vi "Update State.vi"(8 "error in (no error)":errorcluster, 11 "BiStableShutter in":refnum<class "BiStableShutter.lvclass">) -> (0 "error out":errorcluster, 3 "BiStableShutter out":refnum<class "BiStableShutter.lvclass">)   [LabVIEW 2016, in "BiStableShutter.lvclass"]
uses:
  BiStableShutter.lvclass
  Controls/Shutter States.ctl
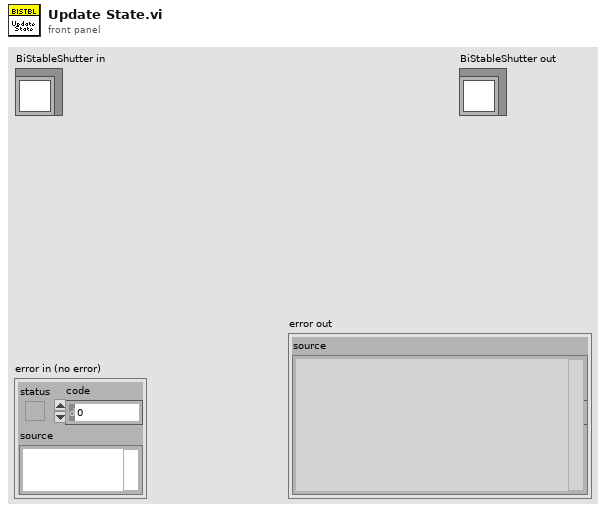
[diagram p1: front panel]
types:
  T1 = typedef "Shutter States.ctl" = enum16{"Open", "Close", "Wait", "Off", "Arm", "Idle"}
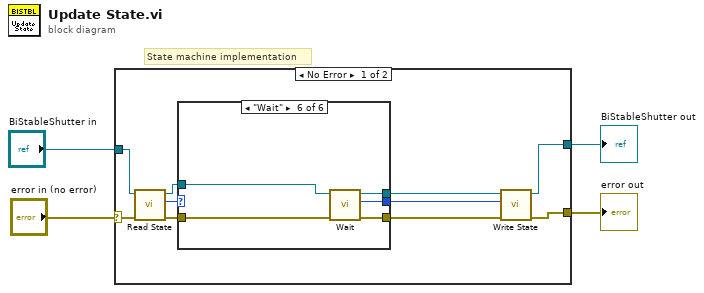
[diagram p0: block diagram]
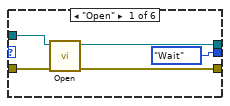
[diagram p2: hidden frame]
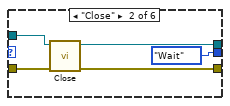
[diagram p3: hidden frame]
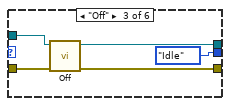
[diagram p4: hidden frame]
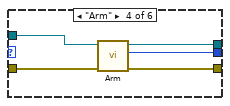
[diagram p5: hidden frame]
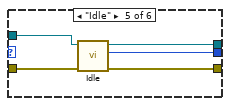
[diagram p6: hidden frame]
diagram:
  # "State machine implementation"
  n1 = case shown="No Error" "error in (no error)" {
    selector: "error in (no error)" -> [w5 w46]
    tunnel: [w14 w45] -> w4
    tunnel: [w12 w46] -> w3
    tunnel: "BiStableShutter in" -> [w9 w45]
    frame No Error {
      n2 = call-dynamic "Read State.vi"("error in (no error)"=w5, "Shutter in"=w9) -> ("error out"=w7:errorcluster, "State"=w6:T1, "Shutter out"=w8:refnum<class "BiStableShutter.lvclass">)  [unwired: 7 in]
      n3 = case shown="\"Wait\"" w6 {
        tunnel: w8 -> [w18 w24 w27 w34 w39 w44]
        tunnel: w7 -> [w19 w23 w29 w30 w38 w43]
        tunnel: [w16 w21 w28 w31 w35 w40] -> w13
        tunnel: [w15 w22 w26 w33 w36 w42] -> w10
        tunnel: [Shutter_States."Wait" ("State") Shutter_States."Wait" ("f") Shutter_States."Idle" ("State") w32 w37 w41] -> w11
        frame "Open" {
          n4 = call-dynamic "Open.vi"("error in (no error)"=w19, "BiStableShutter in"=w18) -> ("error out"=w16:errorcluster, "BiStableShutter out"=w15:refnum<class "BiStableShutter.lvclass">)  [unwired: 8 in]
        }
        frame "Close" {
          n5 = call-dynamic "Close.vi"("error in (no error)"=w23, "BiStableShutter in"=w24) -> ("error out"=w21:errorcluster, "BiStableShutter out"=w22:refnum<class "BiStableShutter.lvclass">)  [unwired: 8 in]
        }
        frame "Off" {
          n6 = call-dynamic "Off.vi"("error in (no error)"=w29, "BiStableShutter in"=w27) -> ("error out"=w28:errorcluster, "BiStableShutter out"=w26:refnum<class "BiStableShutter.lvclass">)  [unwired: 8 in]
        }
        frame "Arm" {
          n7 = call-dynamic "Arm.vi"("error in (no error)"=w30, "Shutter in"=w34) -> ("error out"=w31:errorcluster, "State"=w32:T1, "Shutter out"=w33:refnum<class "BiStableShutter.lvclass">)  [unwired: 7 in]
        }
        frame "Idle" {
          n8 = call-dynamic "Idle.vi"("error in (no error)"=w38, "Shutter in"=w39) -> ("error out"=w35:errorcluster, "State"=w37:T1, "Shutter out"=w36:refnum<class "BiStableShutter.lvclass">)  [unwired: 7 in]
        }
        frame "Wait" {
          n9 = call-dynamic "Wait.vi"("error in (no error)"=w43, "BiStableShutter in"=w44) -> ("error out"=w40:errorcluster, "State"=w41:T1, "BiStableShutter out"=w42:refnum<class "BiStableShutter.lvclass">)  [unwired: 7 in]
        }
      }
      n10 = call-dynamic "Write State.vi"("error in (no error)"=w13, "Set"=w11, "Shutter in"=w10) -> ("error out"=w12:errorcluster, "Shutter out"=w14:refnum<class "BiStableShutter.lvclass">)  [unwired: 7 in]
    }
    frame Error {
    }
  }
  "error out" <- w3
  "BiStableShutter out" <- w4
